vi "ESP300 Goto.vi"(5 "Axe Inv":bool, 6 "Input Units":i8(ring) items=["mm", "ps"], 7 "ESP300Ref":T1, 8 "error in":errorcluster, 9 "Axis":i8(ring)=1 items=["Axis 1"=1, "Axis 2"=2, "Axis 3"=3], 10 "Position":dbl=0.5, 11 "VISA Rsrc":refnum<visa-resource-name>="GPIB0::7::INSTR") -> (0 "error out":errorcluster, 2 "Pos Out":dbl=0.5)   [LabVIEW 2010]
uses:
  <userlib>/ESP300/ESP300 GotoState.ctl
  <userlib>/GenProg/WritebyRefNum.vi
panel:
  out "Move Done":bool
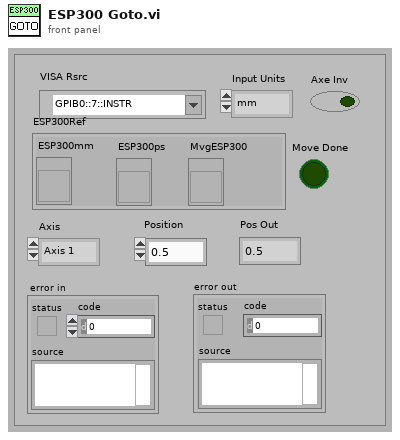
[diagram p1: front panel]
types:
  T1 = cluster{"ESP300mm":refnum<vi>, "ESP300ps":refnum<vi>, "MvgESP300":refnum<vi>}
  T2 = typedef "ESP300 GotoState.ctl" = enum16{"send command", "read position", "check status", "end"}
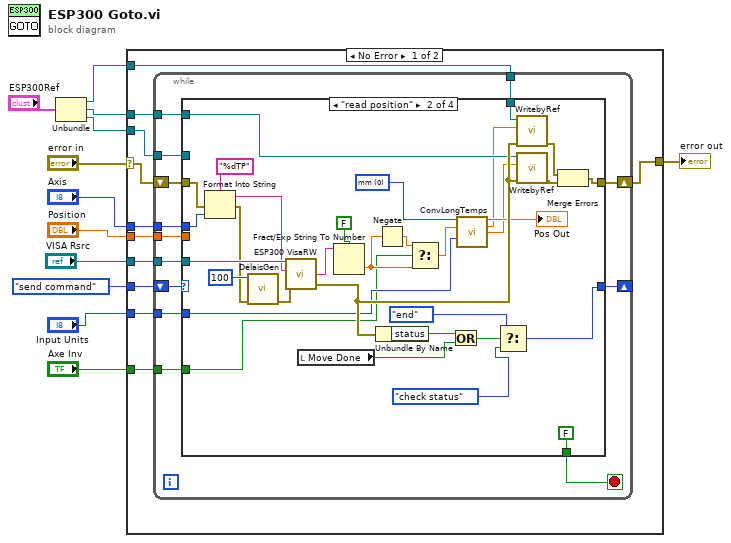
[diagram p0: block diagram]
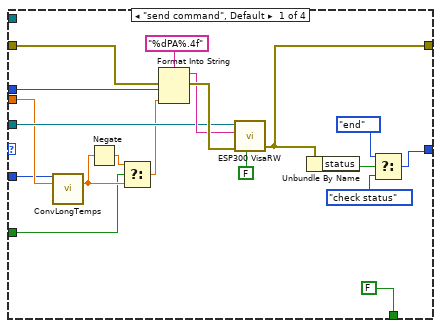
[diagram p2: hidden frame]
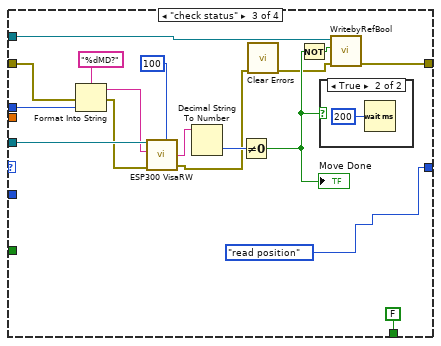
[diagram p3: hidden frame]
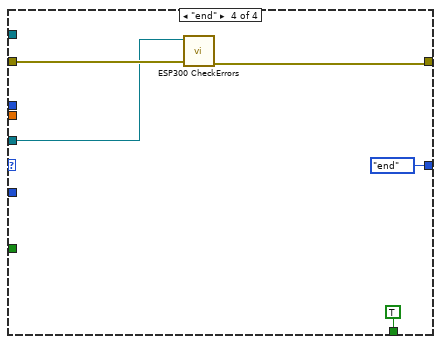
[diagram p5: hidden frame]
diagram:
  n1 = Unbundle("ESP300Ref") -> ("ESP300mm"=w2:refnum<vi>, "ESP300ps"=w4:refnum<vi>, "MvgESP300"=w3:refnum<vi>)
  n2 = case shown="No Error" "error in" {
    selector: "error in" -> [w20 w111]
    tunnel: "Axis" -> [w22 _]
    tunnel: "Position" -> [w23 _]
    tunnel: [w19 w111] -> w9
    tunnel: ESP300_GotoState."send command" ("Énum") -> [w21 _]
    tunnel: "VISA Rsrc" -> [w18 _]
    tunnel: w3 -> [w17 _]
    tunnel: "Input Units" -> [w16 _]
    tunnel: w2 -> [w15 _]
    tunnel: w4 -> [w14 _]
    tunnel: "Axe Inv" -> [w13 _]
    frame No Error {
      n3 = while {
        tunnel: w23 -> [w36]
        tunnel: w22 -> [w35]
        shift-right: [w31] -> w19
        shift-left: w20 -> [w33]
        tunnel: w18 -> [w32]
        shift-right: [w29] -> _
        shift-left: w21 -> [w34]
        tunnel: w17 -> [w28]
        tunnel: w16 -> [w27]
        tunnel: w15 -> [w26]
        tunnel: w14 -> [w25]
        tunnel: w13 -> [w24]
        stop <- w30 stop-if-true
        n4 = case shown="\"read position\"" w34 {
          tunnel: w36 -> [w42 _ _ _]
          tunnel: w35 -> [w54 w85 w102 _]
          tunnel: w33 -> [w53 w84 w101 w108]
          tunnel: w32 -> [w50 w87 w104 w106]
          tunnel: [w47 w68 w92 w107] -> w31
          tunnel: [FALSE FALSE FALSE TRUE] -> w30
          tunnel: [w44 w77 ESP300_GotoState."read position" ("Énum") ESP300_GotoState."end" ("Énum")] -> w29
          tunnel: w28 -> [_ _ w94 _]
          tunnel: w27 -> [w41 w60 _ _]
          tunnel: w26 -> [_ w66 _ _]
          tunnel: w25 -> [_ w65 _ _]
          tunnel: w24 -> [w37 w56 _ _]
          frame "send command", Default {
            n5 = call <userlib>:"ConvLongTemps.vi"("Input Units"=w41, "Units Input"=w42) -> ("Units mm"=w38:dbl)  [unwired: 10 in, 3 out]
            n6 = Negate(x=w38) -> (-x=w39:dbl)
            n7 = Select(t=w39, s=w37, f=w38) -> (s? t:f=w40:dbl)
            n8 = Format Into String(format string="%dPA%.4f", error in=w53, w54, w40) -> (resulting string=w51:string, error out=w52:errorcluster)  [unwired: 1 in]
            n9 = call <userlib>:"ESP300 VisaRW.vi"("Lecture?(T)"=FALSE, "error in (no error)"=w52, "ChaineCom"=w51, "VISA Rsrc"=w50) -> ("error out"=w47:errorcluster)  [unwired: 3 in, 3 out]
            n10 = Unbundle By Name(w47) -> ("status"=w46:bool)
            n11 = Select(t=ESP300_GotoState."end" ("Énum"), s=w46, f=ESP300_GotoState."check status" ("Énum")) -> (s? t:f=w44:T2)
          }
          frame "read position" {
            w64 = i8 0 items=["mm", "ps"] ("Input Units")
            n12 = Format Into String(format string="%dTP", error in=w84, w85) -> (resulting string=w83:string, error out=w72:errorcluster)  [unwired: 1 in]
            n13 = call <userlib>:"DélaisGen.vi"("error in (no error)"=w72, "Numérique"=u32 100 ("milliseconds to wait")) -> ("error out"=w73:errorcluster)  [unwired: 9 in]
            n14 = call <userlib>:"ESP300 VisaRW.vi"("error in (no error)"=w73, "ChaineCom"=w83, "VISA Rsrc"=w87) -> ("error out"=w69:errorcluster, "ChaineRep"=w82:string)  [unwired: 4 in, 2 out]
            n15 = local read "Move Done"() -> (w71:bool)
            n16 = Fract/Exp String To Number(use system decimal point (T)=FALSE ("utiliser le séparateur décimal du système (V)"), string=w82) -> (number=w58:dbl)  [unwired: 2 in, 1 out]
            n17 = Unbundle By Name(w69) -> ("status"=w76:bool)
            n18 = Negate(x=w58) -> (-x=w59:dbl)
            n19 = Select(t=w59, s=w56, f=w58) -> (s? t:f=w57:dbl)
            n20 = Or(x=w76, y=w71) -> (x .or. y?=w75:bool)
            n21 = call <userlib>:"ConvLongTemps.vi"("Input Units"=w64, "Units Input"=w57, "Output Units"=w60) -> ("Units Output"=→"Pos Out":dbl, "Units mm"=w62:dbl, "Units ps"=w61:dbl)  [unwired: 9 in, 1 out]
            n22 = Select(t=ESP300_GotoState."end" ("Énum"), s=w75, f=ESP300_GotoState."check status" ("Énum")) -> (s? t:f=w77:T2)
            n23 = call-poly <userlib>:"WritebyRef.vi"("error in"=w69, "Valeur"=w62, "Control Ref"=w66) -> ("error out"=w67:errorcluster)  [unwired: 8 in]
            n24 = call-poly <userlib>:"WritebyRef.vi"("error in"=w69, "Valeur"=w61, "Control Ref"=w65) -> ("error out"=w70:errorcluster)  [unwired: 8 in]
            n25 = Merge Errors(w67, w70) -> (w68:errorcluster)
          }
          frame "check status" {
            n26 = Format Into String(format string="%dMD?", error in=w101, w102) -> (resulting string=w99:string, error out=w100:errorcluster)  [unwired: 1 in]
            n27 = call <userlib>:"ESP300 VisaRW.vi"("Délais (0 ms)"=u32 100, "error in (no error)"=w100, "ChaineCom"=w99, "VISA Rsrc"=w104) -> ("error out"=w93:errorcluster, "ChaineRep"=w98:string)  [unwired: 3 in, 2 out]
            n28 = Decimal String To Number(string=w98) -> (number=w96:i32)  [unwired: 2 in, 1 out]
            n29 = Not Equal To 0?(x=w96) -> (x != 0?=w91:bool)
            "Move Done" <- w91
            n30 = call <vilib>:"Clear Errors.vi"("error in (no error)"=w93) -> ("error out"=w88:errorcluster)  [unwired: 6 in]
            n31 = Not(x=w91) -> (.not. x?=w90:bool)
            n32 = case shown="True" w91 {
              frame False {
              }
              frame True {
                n33 = Wait (ms)(milliseconds to wait=u32 200) -> ()  [unwired: 1 out]
              }
            }
            n34 = call <userlib>:"WritebyRefBool.vi"("error in"=w88, "Valeur"=w90, "Control Ref"=w94) -> ("error out"=w92:errorcluster)  [unwired: 8 in]
          }
          frame "end" {
            n35 = call <userlib>:"ESP300 CheckErrors.vi"("error in (no error)"=w108, "Ressource VISA In"=w106) -> ("error out"=w107:errorcluster)  [unwired: 4 in, 3 out]
          }
        }
      }
    }
    frame Error {
    }
  }
  "error out" <- w9
